vi "Image Compression.vi"() -> ()   [LabVIEW 2023]
doc: "This example shows the application of the discrete wavelet transform (DWT) in image compression.\n\nThe DWT transforms an image into wavelet coefficients. The wavelet coefficients have most values close to zero. After quantizing the wavelet coefficients, you can set most of the coefficients to zero. So you can use entropy-based encoding techniques to reduce the bit rate of the wavelet coefficients and achieve image compression.\n\nThis example uses the WA Discrete Wavelet Transform VI to transform an image into wavelet coefficients and simulates the quantization for the wavelet coefficients. From the quantized wavelet coefficients, this example reconstructs the image using the WA Inverse Discrete Wavelet Transform VI and computes the peak signal to noise ratio (PSNR) of the reconstructed image. In real-world image compression applications, you achieve compression by using entropy-based encoding techniques such as the Huffman coding to encode the quantized wavelet coefficients.\n\n<b>Instructions:</b>\n1) Run this VI.\n2) Change the number of <b>Bits</b> to quantize the wavelet transform and observe the <b>PSNR (dB)</b> of the image."
uses:
  <vilib>/addons/Wavelet Analysis/discrete wavelet transform.llb/WA 2D Discrete Wavelet Transform.vi
  <vilib>/addons/Wavelet Analysis/discrete wavelet transform.llb/WA Inverse 2D Discrete Wavelet Transform.vi
  <vilib>/addons/_Advanced Signal Processing/NI_AdvSigProcWA.lvlib
panel:
  in  "Image":u16(ring)=122 items=["Finger Print (Image)"=121, "Iris Flower (Image)"=122, "Mammogram (Image)"=123, "Lake (Image)"=127, "Two Can 1 (Image)"=132, "Two Can 2 (Image)"=133, "Camera Man (Image)"=134]
  in  "stop":bool
  out "PSNR (dB)":dbl=35.634693516588186
  out "Reconstructed Image":dbl[][](graph)
  out "Original Image":u8[][](graph)
  in  "Bits":i32=8 min=1 max=64
  in  "Wavelet":u16(ring) items=["db02"=0, "db03"=1, "db04"=2, "db05"=3, "db06"=4, "db07"=5, "db08"=6, "db09"=7, "db10"=8, "db11"=9, "db12"=10, "db13"=11, "db14"=12, "Haar"=13, "bior1_3"=14, "bior1_5"=15, "bior2_2"=16, "bior2_4"=17, "bior2_6"=18, "bior2_8"=19, "bior3_1"=20, "bior3_3"=21, "bior3_5"=22, "bior3_7"=23, "bior3_9"=24, "bior4_4 (FBI)"=25, "bior5_5"=38, "bior6_8"=39, "coif1"=26, "coif2"=27, "coif3"=28, "coif4"=29, "coif5"=30, "sym2"=31, "sym3"=32, "sym4"=33, "sym5"=34, "sym6"=35, "sym7"=36, "sym8"=37]
  in  "Levels":i32=8
  # "Overview: Shows the application of the discrete wavelet transform (DWT) in image compression.\nRequirements: LabVIEW Full Development System, Advanced Signal Processing Toolkit\nInstructions: \n1. Run this VI.\n2. Change the number of Bits to quantize the wavelet transform and observe the PSNR (dB) of the image.\n3. Click Stop to stop the VI."
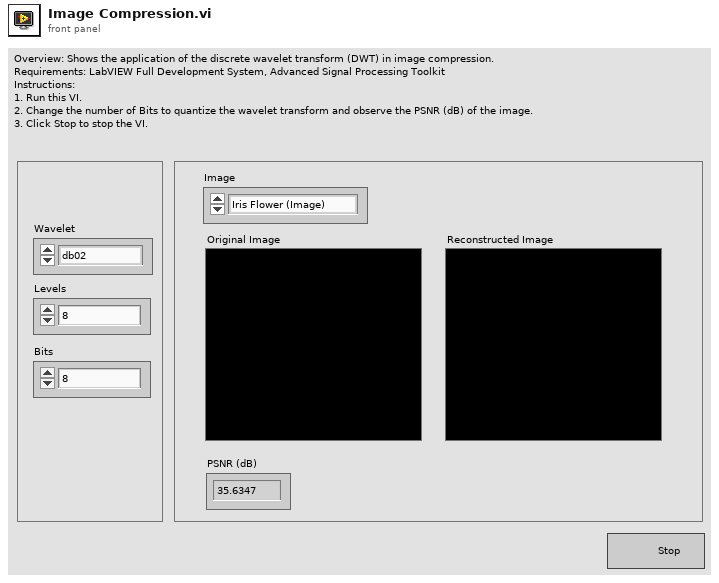
[diagram p1: front panel]
types:
  T1 = cluster{"low_low":dbl[][], "low_high":dbl[][], "high_low":dbl[][], "high_high":dbl[][]}[]
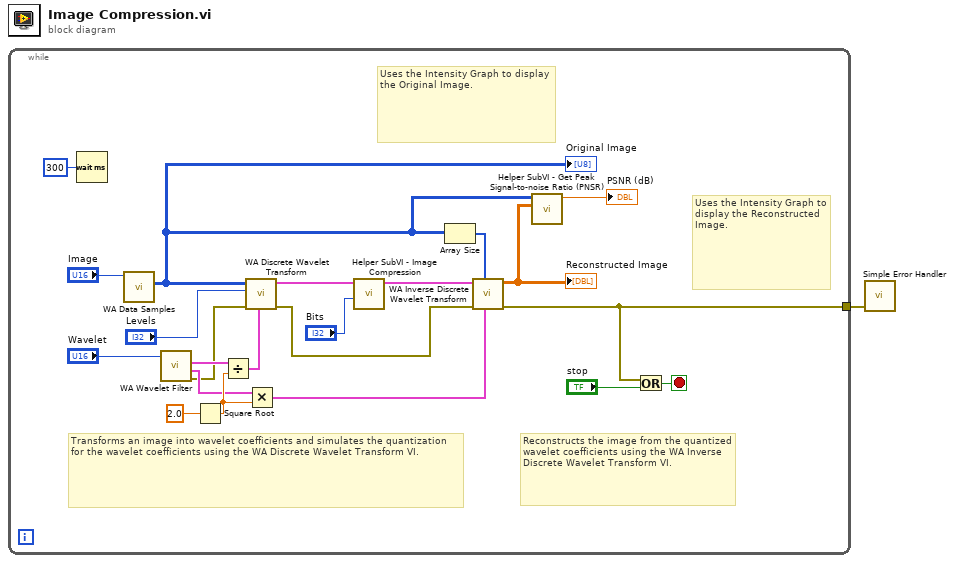
[diagram p0: block diagram]
diagram:
  n1 = while {
    tunnel: [w7] -> w1
    stop <- w10 stop-if-true
    # "Uses the Intensity Graph to display the Reconstructed Image."
    # "Uses the Intensity Graph to display the Original Image."
    # "Reconstructs the image from the quantized wavelet coefficients using the WA Inverse Discrete Wavelet Transform VI."
    # "Transforms an image into wavelet coefficients and simulates the quantization for the wavelet coefficients using the WA Discrete Wavelet Transform VI."
    n2 = Wait (ms)(milliseconds to wait=u32 300 ("millisecond multiple")) -> ()  [unwired: 1 out]
    n3 = call <vilib>:"WA Data Samples.vi"("data"="Image") -> ("image"=w4:u8[][])  [unwired: 10 out]
    "Original Image" <- w4
    n4 = call <vilib>:"WA Wavelet Filter.vi"("wavelet"="Wavelet") -> ("error out"=w6:errorcluster, "synthesis filters"=w12:cluster{"lowpass":dbl[], "highpass":dbl[]}, "analysis filters"=w18:cluster{"lowpass":dbl[], "highpass":dbl[]})  [unwired: 3 in, 5 out]
    n5 = Square Root(x=2.0) -> (sqrt(x)=w13:dbl)
    n6 = Divide(x=w18, y=w13) -> (x/y=w15:cluster{"lowpass":dbl[], "highpass":dbl[]})
    n7 = call-poly <vilib>:"WA Discrete Wavelet Transform.vi"("analysis filters"=w15, "error in (no error)"=w6, "levels"="Levels", "signal"=w4) -> ("error out"=w5:errorcluster, "DWT coef"=w21:T1)  [unwired: 1 in, 5 out]
    n8 = Multiply(x=w12, y=w13) -> (x*y=w14:cluster{"lowpass":dbl[], "highpass":dbl[]})
    n9 = call "Helper SubVI - Image Compression.vi"("bits"="Bits", "2D DWT coef"=w21) -> ("compressed coef"=w20:T1)  [unwired: 9 out]
    n10 = Array Size(array=w4) -> (size(s)=w19:i32[])
    n11 = call-poly <vilib>:"WA Inverse Discrete Wavelet Transform.vi"("synthesis filters"=w14, "size"=w19, "error in (no error)"=w5, "DWT coef"=w20) -> ("error out"=w7:errorcluster, "signal"=w3:dbl[][])  [unwired: 1 in, 5 out]
    "Reconstructed Image" <- w3
    n12 = call "Helper SubVI - Get Peak Signal-to-noise Ratio (PNSR).vi"("dest"=w3, "source"=w4) -> ("PSNR (dB)"=→"PSNR (dB)":dbl)  [unwired: 9 in]
    n13 = Or(x=w7, y="stop") -> (x .or. y?=w10:bool)
  }
  n14 = call <vilib>:"Simple Error Handler.vi"("error in (no error)"=w1) -> ()  [unwired: 1 in, 8 out]
